vi "Periodic Tasks.vi"(8 "error in":errorcluster) -> ()   [LabVIEW 2019]
doc: "This VI runs in parallel to other tasks. It can contain as many user-defined periodic loops as you need. These can carry out PID or other sorts of timed response."
uses:
  Robot Global Data.vi
  <vilib>/Rock Robotics/Network Tables/NT Read Number.vi
  <vilib>/Rock Robotics/Network Tables/NT Write Number.vi
  <vilib>/Rock Robotics/Network Tables/NT Write String.vi
panel:
  in  "Setpoint":dbl
  out "Color":u32(colorbox)
  out "Measured Color":cluster{"R":dbl, "G":dbl, "B":dbl}
  out "Match Confidence":dbl
  out "Matched Color Name":string
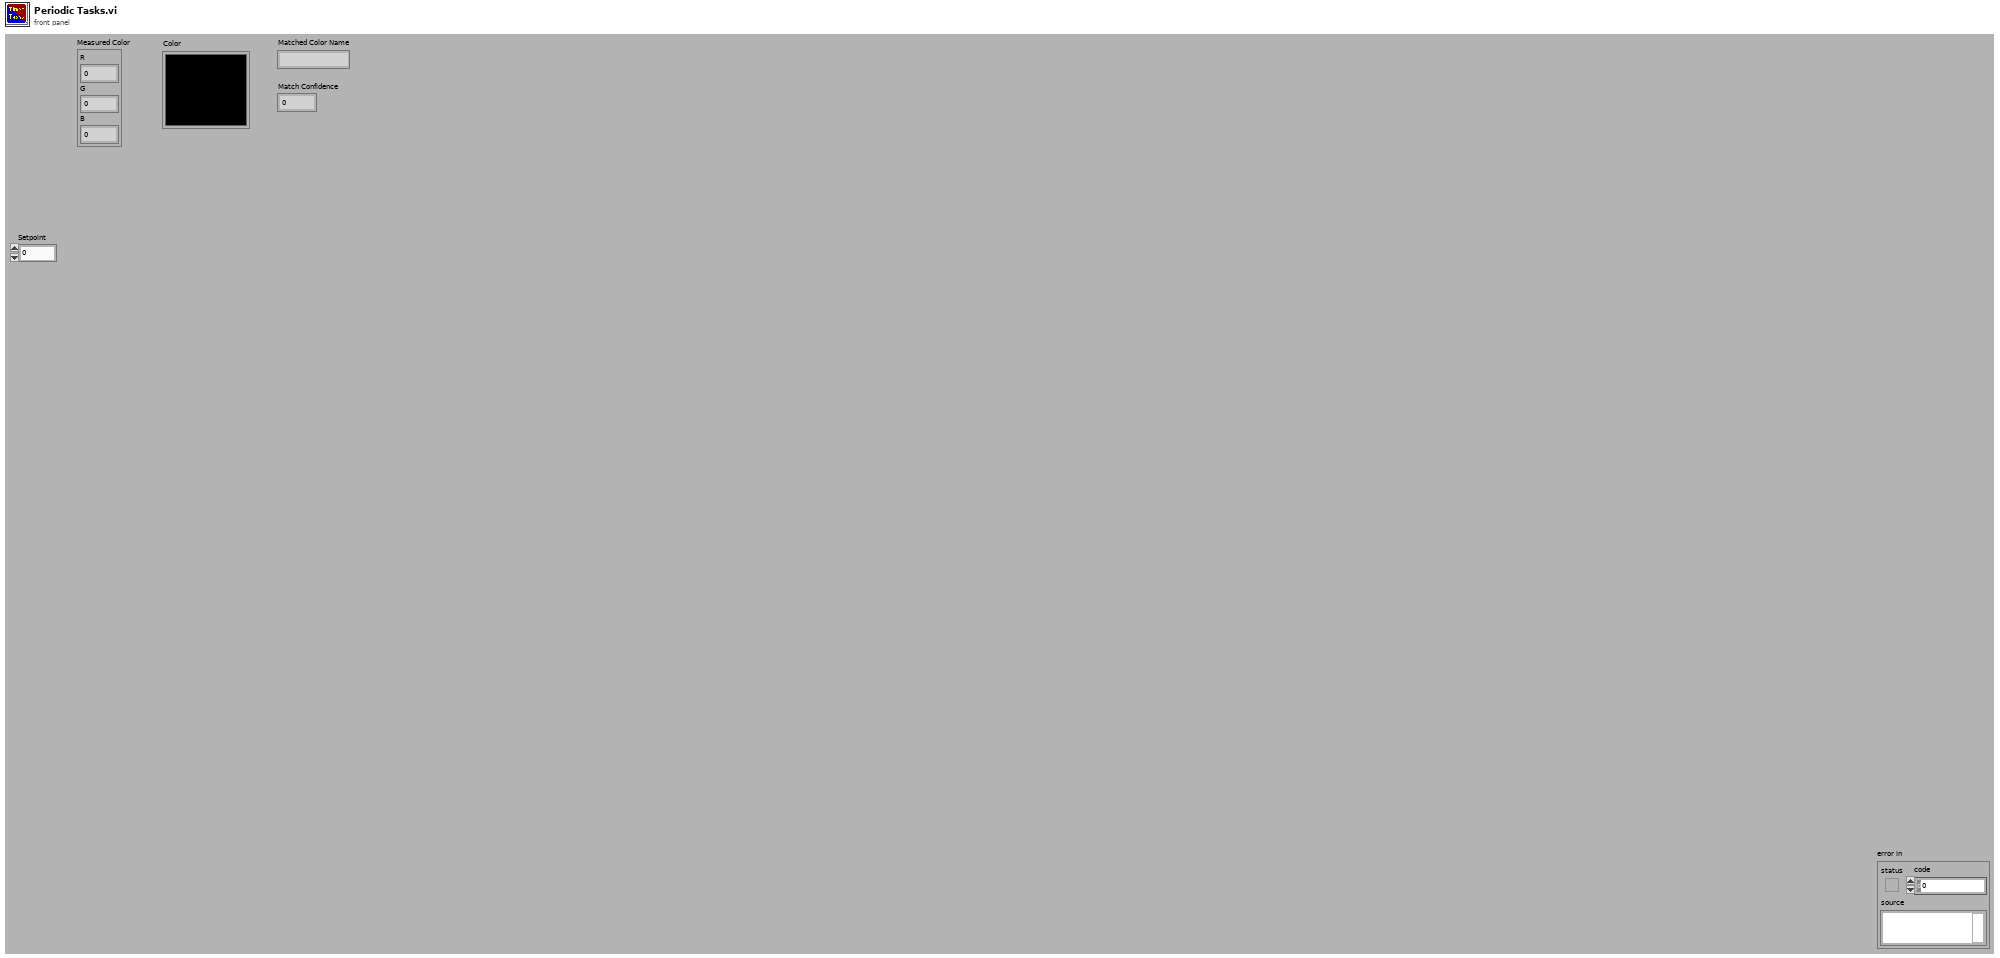
[diagram p1: front panel]
types:
  T1 = typedef "WPI_GyroDevRef.ctl" = cluster{"DevStatus":errorcluster, "Analog Channel":T2, "Gain (VoltsPerDegree/Second)":dbl, "Gyro Type":enum16{"Analog", "XRS450"}, "Handle":i32, "SPI Bus":T3, "Device Found":bool, "Sample Rate":dbl, "Calibrate On Open":bool, "Offset":dbl}
  T2 = typedef "FPGA_AIChannel.ctl" = enum8{"AI 0", "AI 1", "AI 2", "AI 3", "AI MXP 0", "AI MXP 1", "AI MXP 2", "AI MXP 3", "Invalid"}
  T3 = typedef "spi_bus.ctl" = enum16{"SPI On-Board, CS0", "SPI On-Board, CS1", "SPI On-Board, CS2", "SPI On-Board, CS3", "SPI MXP", "Invalid"}
  T4 = typedef "WPI_DigitalInputDevRef.ctl" = cluster{"DevStatus":errorcluster, "DIO Channel":T5}
  T5 = typedef "FPGA_DIOChannel.ctl" = enum8{"DIO 0", "DIO 1", "DIO 2", "DIO 3", "DIO 4", "DIO 5", "DIO 6", "DIO 7", "DIO 8", "DIO 9", "DIO MXP 0", "DIO MXP 1", "DIO MXP 2", "DIO MXP 3", "DIO MXP 4", "DIO MXP 5", "DIO MXP 6", "DIO MXP 7", "DIO MXP 8", "DIO MXP 9", "DIO MXP 10", "DIO MXP 11", "DIO MXP 12", "DIO MXP 13", "DIO MXP 14", "DIO MXP 15", "SPI Port CS1", "SPI Port CS2", "SPI Port CS3", "SPI Port MISO", "SPI Port MOSI", "Invalid"}
  T6 = typedef "WPI_JoystickDevRef.ctl" = cluster{"Device":T7}
  T7 = typedef "WPI_JoystickDeviceEnum.ctl" = enum16{"USB 0", "USB 1", "USB 2", "USB 3", "USB 4", "USB 5"}
  T8 = typedef "WPI_RobotDriveDevRef.ctl" = cluster{"DevStatus":errorcluster, "Motors[]":T9[], "Square Inputs":bool, "Max Output":dbl}
  T9 = typedef "WPI_MotorControlDeviceRef.ctl" = cluster{"DeviceStatus":errorcluster, "Type":T10, "PWM":cluster{"PWM Channel":T11, "DeadBand":T12}, "CAN":cluster{"Device Number":u8, "SetOutput VI Ref":variant, "GetOutput VI Ref":variant, "Enable VI Ref":variant, "Disable VI Ref":variant, "Data":variant}, "Invert":bool, "DIO PWM":cluster{"PWM \"Enable\" Channel":T11, "DIOChannel":T5, "PWM Rate":dbl}}
  T10 = typedef "WPI_MotorControlType.ctl" = enum16{"PWM", "CAN", "DIO PWM"}
  T11 = typedef "FPGA_DIOPWMChannel.ctl" = enum8{"PWM 0", "PWM 1", "PWM 2", "PWM 3", "PWM 4", "PWM 5", "PWM 6", "PWM 7", "PWM 8", "PWM 9", "PWM MXP 0", "PWM MXP 1", "PWM MXP 2", "PWM MXP 3", "PWM MXP 4", "PWM MXP 5", "PWM MXP 6", "PWM MXP 7", "PWM MXP 8", "PWM MXP 9", "Invalid"}
  T12 = typedef "WPI_PWMDeadband.ctl" = cluster{"Name":string, "maxPositivePwm":i32, "minPositivePwm":i32, "centerPwm":i32, "maxNegativePwm":i32, "minNegativePwm":i32, "angularRange":u16}
  T13 = cluster{"JoystickDevRef":T6, "RobotDriveDevRef":T8}
  T14 = typedef "Color Sensor V3 DevRef.ctl" = cluster{"I2CDevRef":T15}
  T15 = typedef "WPI_I2CDevRef.ctl" = cluster{"DevStatus":errorcluster, "Device Address":u8, "Handle":i32, "I2C Bus":T16}
  T16 = typedef "i2c_bus.ctl" = enum16{"I2C On-Board", "I2C MXP", "Invalid"}
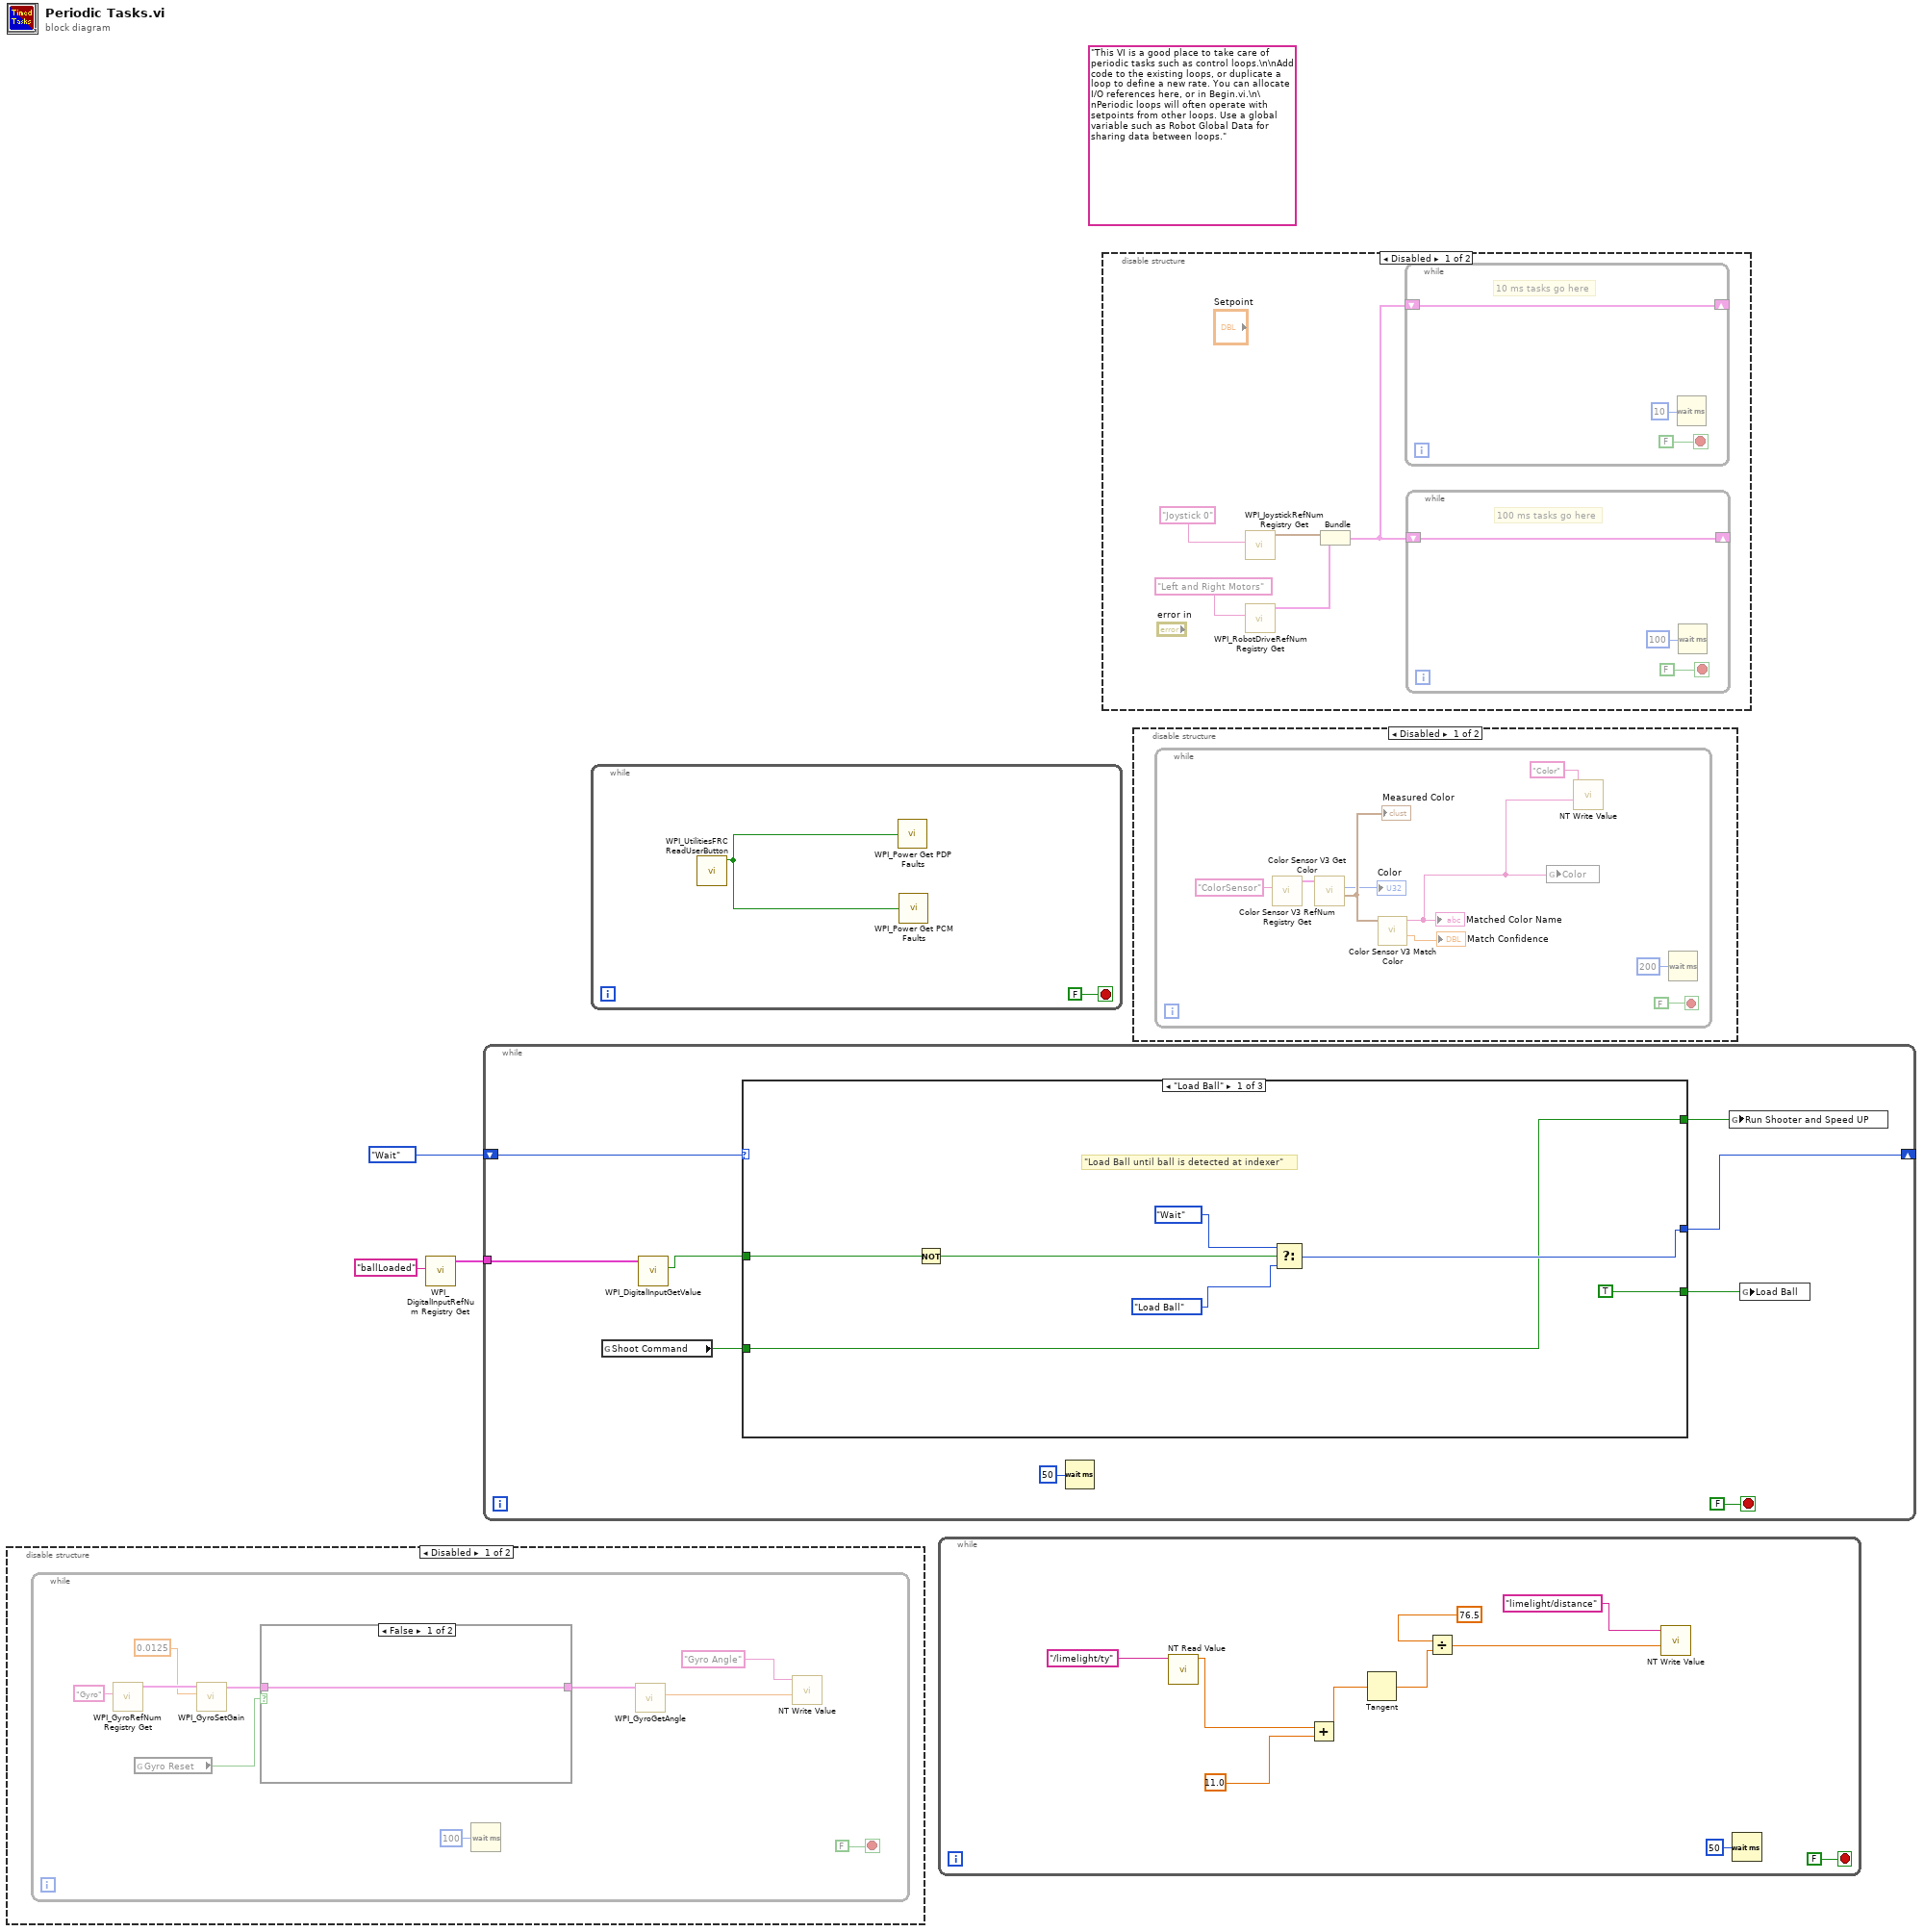
[diagram p0: block diagram]
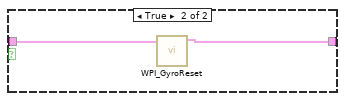
[diagram p3: hidden frame]
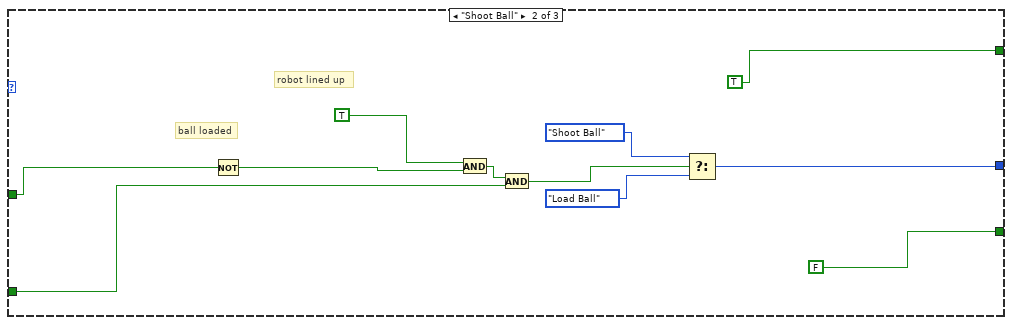
[diagram p5: hidden frame]
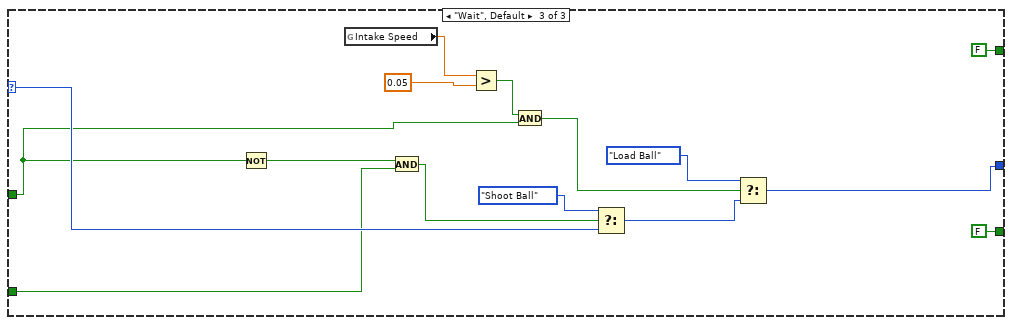
[diagram p6: hidden frame]
diagram:
  (unwired) "This VI is a good place to take care of periodic tasks such as control loops.\n\nAdd code to the existing loops, or duplicate a loop to define a new rate. You can allocate I/O references here, or in Begin.vi.\n\nPeriodic loops will often operate with setpoints from other loops. Use a global variable such as Robot Global Data for sharing data between loops."
  n1 = disable-structure shown="Disabled" {
    frame Disabled {
      n2 = while {
        stop <- FALSE stop-if-true
        n3 = call <vilib>:"WPI_GyroRefNum Registry Get.vi"("refnum name"="Gyro") -> ("GyroDevRef"=w7:T1)  [unwired: 9 in, 1 out]
        n4 = global read "Robot Global Data.vi" "Gyro Reset"() -> (w9:bool)
        n5 = call <vilib>:"WPI_GyroSetGain.vi"("Gain (VoltsPerDegree/Second)"=0.0125, "GyroDevRef"=w7) -> ("GyroDevRef"=w8:T1)  [unwired: 8 in, 1 out]
        n6 = case shown="False" w9 {
          tunnel: w8 -> [w14 w16]
          tunnel: [w14 w15] -> w13
          frame False {
          }
          frame True {
            n7 = call <vilib>:"WPI_GyroReset.vi"("GyroDevRef"=w16) -> ("GyroDevRef"=w15:T1)  [unwired: 9 in, 1 out]
          }
        }
        n8 = Wait (ms)(milliseconds to wait=u32 100) -> ()  [unwired: 1 out]
        n9 = call <vilib>:"WPI_GyroGetAngle.vi"("GyroDevRef"=w13) -> ("Angle"=w11:dbl)  [unwired: 6 in, 4 out]
        n10 = call-poly <vilib>:"NT Write Value.vi"("Numeric"=w11, "Name"="Gyro Angle") -> ()  [unwired: 9 in, 1 out]
      }
    }
    frame Enabled {
    }
  }
  n11 = call <vilib>:"WPI_DigitalInputRefNum Registry Get.vi"("refnum name"="ballLoaded") -> ("DigitalInputDevRef"=w2:T4)  [unwired: 9 in, 1 out]
  n12 = while {
    shift-right: [w24] -> _
    shift-left: enum16{"Wait", "Load Ball", "Shoot Ball"}."Wait" -> [w25]
    tunnel: w2 -> [w19]
    stop <- FALSE stop-if-true
    n13 = global read "Robot Global Data.vi" "Shoot Command"() -> (w17:bool)
    n14 = call <vilib>:"WPI_DigitalInputGetValue.vi"("DigitalInputDevRef"=w19) -> ("Value"=w18:bool)  [unwired: 8 in, 2 out]
    n15 = case shown="\"Load Ball\"" w25 {
      selector: w25 -> [_ _ w52]
      tunnel: [w32 w43 w58] -> w24
      tunnel: [TRUE ("Load Ball") FALSE ("Load Ball") FALSE ("Load Ball")] -> w21
      tunnel: [w26 TRUE ("Shoot Ball") FALSE ("Shoot Ball")] -> w20
      tunnel: w18 -> [w27 w36 w45]
      tunnel: w17 -> [w26 w33 w44]
      frame "Load Ball" {
        # "\"Load Ball until ball is detected at indexer\""
        n16 = Not(x=w27) -> (.not. x?=w28:bool)
        n17 = Select(t=enum16{"Wait", "Load Ball", "Shoot Ball"}."Wait", s=w28, f=enum16{"Wait", "Load Ball", "Shoot Ball"}."Load Ball") -> (s? t:f=w32:enum16{"Wait", "Load Ball", "Shoot Ball"})
      }
      frame "Shoot Ball" {
        # "ball loaded"
        # "robot lined up"
        n18 = Not(x=w36) -> (.not. x?=w37:bool)
        n19 = And(x=TRUE, y=w37) -> (x .and. y?=w35:bool)
        n20 = And(x=w35, y=w33) -> (x .and. y?=w34:bool)
        n21 = Select(t=enum16{"Wait", "Load Ball", "Shoot Ball"}."Shoot Ball", s=w34, f=enum16{"Wait", "Load Ball", "Shoot Ball"}."Load Ball") -> (s? t:f=w43:enum16{"Wait", "Load Ball", "Shoot Ball"})
      }
      frame "Wait", Default {
        n22 = Not(x=w45) -> (.not. x?=w46:bool)
        n23 = global read "Robot Global Data.vi" "Intake Speed"() -> (w54:dbl)
        n24 = And(x=w46, y=w44) -> (x .and. y?=w49:bool)
        n25 = Greater?(x=w54, y=0.05) -> (0:w47:bool)
        n26 = And(x=w47, y=w45) -> (x .and. y?=w48:bool)
        n27 = Select(t=enum16{"Wait", "Load Ball", "Shoot Ball"}."Shoot Ball", s=w49, f=w52) -> (s? t:f=w57:enum16{"Wait", "Load Ball", "Shoot Ball"})
        n28 = Select(t=enum16{"Wait", "Load Ball", "Shoot Ball"}."Load Ball", s=w48, f=w57) -> (s? t:f=w58:enum16{"Wait", "Load Ball", "Shoot Ball"})
      }
    }
    n29 = Wait (ms)(milliseconds to wait=u32 50) -> ()  [unwired: 1 out]
    n30 = global write "Robot Global Data.vi" "Run Shooter and Speed UP"(w20) -> ()
    n31 = global write "Robot Global Data.vi" "Load Ball"(w21) -> ()
  }
  n32 = while {
    stop <- FALSE stop-if-true
    n33 = call <vilib>:"WPI_UtilitiesFRC ReadUserButton.vi"() -> ("User Button"=w59:bool)  [unwired: 10 in, 1 out]
    n34 = call <vilib>:"WPI_Power Get PDP Faults.vi"("Clear Sticky Faults"=w59) -> ()  [unwired: 10 in, 5 out]
    n35 = call <vilib>:"WPI_Power Get PCM Faults.vi"("Clear Sticky Faults"=w59) -> ()  [unwired: 11 in, 4 out]
  }
  n36 = while {
    stop <- FALSE stop-if-true
    n37 = call-poly <vilib>:"NT Read Value.vi"("Name"="/limelight/ty") -> ("Numeric"=w64:dbl)  [unwired: 9 in, 1 out]
    n38 = Add(x=w64, y=11.0) -> (x+y=w65:dbl)
    n39 = Tangent(1:w65) -> (0:w66:dbl)
    n40 = Divide(x=76.5, y=w66) -> (x/y=w62:dbl)
    n41 = call-poly <vilib>:"NT Write Value.vi"("Numeric"=w62, "Name"="limelight/distance") -> ()  [unwired: 9 in, 1 out]
    n42 = Wait (ms)(milliseconds to wait=u32 50) -> ()  [unwired: 1 out]
  }
  n43 = disable-structure shown="Disabled" {
    frame Disabled {
      n44 = call <vilib>:"WPI_JoystickRefNum Registry Get.vi"("refnum name"="Joystick 0") -> ("JoystickDevRef"=w73:T6)  [unwired: 1 in, 9 out]
      n45 = call <vilib>:"WPI_RobotDriveRefNum Registry Get.vi"("refnum name"="Left and Right Motors") -> ("RobotDriveDevRef"=w72:T8)  [unwired: 1 in, 9 out]
      n46 = Bundle("JoystickDevRef"=w73, "RobotDriveDevRef"=w72) -> (w71:T13)  [unwired: 1 out]
      n47 = while {
        shift-right: [w79] -> _
        shift-left: w71 -> [w79]
        stop <- FALSE stop-if-true
        # "10 ms tasks go here"
        n48 = Wait (ms)(milliseconds to wait=u32 10) -> ()  [unwired: 1 out]
      }
      n49 = while {
        shift-right: [w76] -> _
        shift-left: w71 -> [w76]
        stop <- FALSE stop-if-true
        # "100 ms tasks go here"
        n50 = Wait (ms)(milliseconds to wait=u32 100) -> ()  [unwired: 1 out]
      }
    }
    frame Enabled {
    }
  }
  n51 = disable-structure shown="Disabled" {
    frame Disabled {
      n52 = while {
        stop <- FALSE stop-if-true
        n53 = call <vilib>:"Color Sensor V3 RefNum Registry Get.vi"("refnum name"="ColorSensor") -> ("ColorSensorDevRef"=w86:T14)  [unwired: 9 in, 1 out]
        n54 = call <vilib>:"Color Sensor V3 Get Color.vi"("ColorSensorDevRef"=w86) -> ("Normalized Color"=w88:cluster{"R":dbl, "G":dbl, "B":dbl}, "Color"=→"Color":u32)  [unwired: 7 in, 2 out]
        "Measured Color" <- w88
        n55 = call <vilib>:"Color Sensor V3 Match Color.vi"("Measured Color"=w88) -> ("Confidence"=→"Match Confidence":dbl, "Matched Color Name"=w83:string)  [unwired: 8 in, 1 out]
        "Matched Color Name" <- w83
        n56 = global write "Robot Global Data.vi" "Color"(w83) -> ()
        n57 = call-poly <vilib>:"NT Write Value.vi"("String"=w83, "Name"="Color") -> ()  [unwired: 9 in, 1 out]
        n58 = Wait (ms)(milliseconds to wait=u32 200) -> ()  [unwired: 1 out]
      }
    }
    frame Enabled {
    }
  }
